vi "GetObjectConfiguration.vi"(8 "ErrorIn":errorcluster, 9 "DataIn":variant, 10 "Label":string, 11 "IApplicationStructureIn":refnum<class "IApplicationConfiguration.lvclass">) -> (0 "ErrorOut":errorcluster, 1 "DataOut":variant, 3 "IApplicationStructureOut":refnum<class "IApplicationConfiguration.lvclass">)   [LabVIEW 2021, in "IApplicationConfiguration.lvclass"]
uses:
  IApplicationConfiguration.lvclass
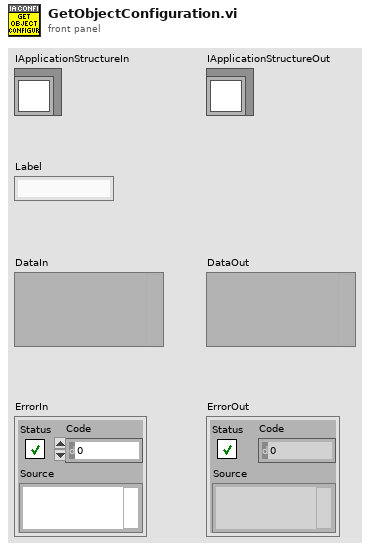
[diagram p1: front panel]
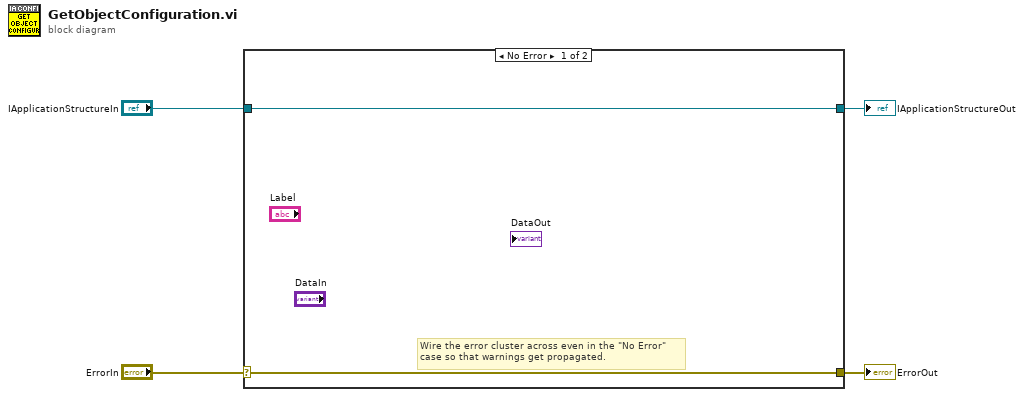
[diagram p0: block diagram]
diagram:
  n1 = case shown="No Error" "ErrorIn" {
    selector: "ErrorIn" -> [w6 w8]
    tunnel: [w6 w8] -> w3
    tunnel: [w5 w7] -> w1
    tunnel: "IApplicationStructureIn" -> [w5 w7]
    frame No Error {
      # "Wire the error cluster across even in the \"No Error\"\ncase so that warnings get propagated."
    }
    frame Error {
    }
  }
  "ErrorOut" <- w3
  "IApplicationStructureOut" <- w1
